vi "get fgpa resources.vi"(8 "error in (no error)":errorcluster, 11 "Item Ref in":T1 format="%.0x") -> (0 "error out":errorcluster, 1 "Found?":bool, 2 "get fpga resources":T2[](array[typedef]), 3 "Item Ref out":T1 format="%.0x")   [LabVIEW 2016, in "FPGA RM Client API.lvlib"]
uses:
  FPGA RM Client API.lvlib
  fpga resource.ctl
  System Explorer/SubVIs/Channel Type.ctl
  <vilib>/NI Veristand/Custom Device API/Custom Device Item Ref.ctl
  <vilib>/NI Veristand/Custom Device API/Get Item Property (Variant).vi
  <vilib>/NI VeriStand/Custom Device API/Custom Device API.lvlib
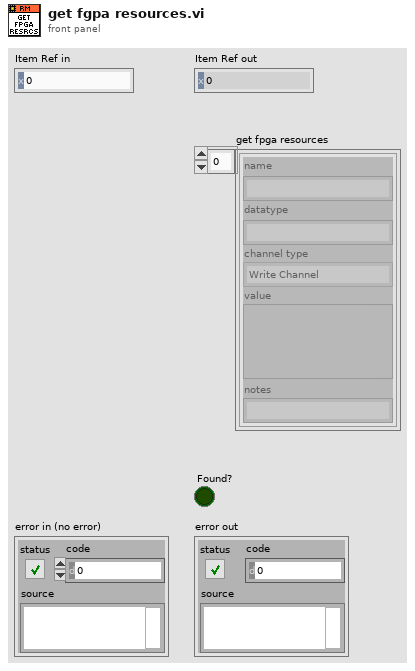
[diagram p1: front panel]
types:
  T1 = typedef "Custom Device API.lvlib/Custom Device Item Ref.ctl" = u64
  T2 = typedef "FPGA RM Client API.lvlib/fpga resource.ctl" = cluster{"name":string, "datatype":string, "channel type":T3, "value":variant, "notes":string}
  T3 = typedef "FPGA RM Client API.lvlib/Channel Type.ctl" = enum16{"Write Channel", "Read Channel", "Write Waveform", "Read Waveform"}
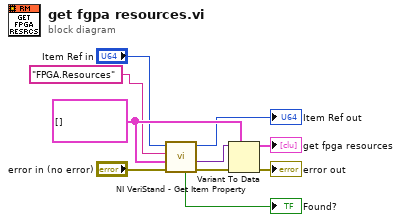
[diagram p0: block diagram]
diagram:
  w7 = T2[] [] ("Array")
  n1 = call-poly <vilib>:"NI VeriStand - Get Item Property.vi"("error in (no error)"="error in (no error)", "Default Value"=w7, "Property Name"="FPGA.Resources" ("string"), "Item Ref in"="Item Ref in") -> ("error out"=w8:errorcluster, "Value"=w6:variant, "Item Ref out"=→"Item Ref out":T1, "Found?"=→"Found?":bool)  [unwired: 4 in]
  n2 = Variant To Data(error in=w8, type=w7, Variant=w6) -> (data=→"get fpga resources":T2[], error out=→"error out":errorcluster)
